vi "E14 BBB Test.vi"(8 "Error In":errorcluster, 11 "Install LV Data":T1={"SSH Session"=refnum, "Status Log"="", "Detailed Log"="", "Credentials"={"Hostname or IP"="192.168.7.2", "Username"="root", "Password"=""}, "Target Info"={"OS Version"="", "CPU"="", "Systemd Version"="", "Internet Access"=FALSE, "Device Type"="", "LV Installed Ver"="", "LV Available Ver"="", "LV Upgrade Available"=FALSE, "Hostname"="", "NIC Info"=[]}, "Reboot Required?"=FALSE}) -> (0 "Error Out":errorcluster, 1 "Status":string, 3 "Install LV Data":T1={"SSH Session"=refnum, "Status Log"="", "Detailed Log"="", "Credentials"={"Hostname or IP"="192.168.7.2", "Username"="root", "Password"=""}, "Target Info"={"OS Version"="", "CPU"="", "Systemd Version"="", "Internet Access"=FALSE, "Device Type"="", "LV Installed Ver"="", "LV Available Ver"="", "LV Upgrade Available"=FALSE, "Hostname"="", "NIC Info"=[]}, "Reboot Required?"=FALSE})   [LabVIEW 2020, in "LMH-LINX.lvlib"]
uses:
  LMH-LINX.lvlib
  Target Management/Install LV Data.ctl
  Target Management/Target Info.ctl
  Target Management/NIC Info.ctl
  Target Management/NIC Mode.ctl
  Toolbox/LMH-Toolbox.lvlib
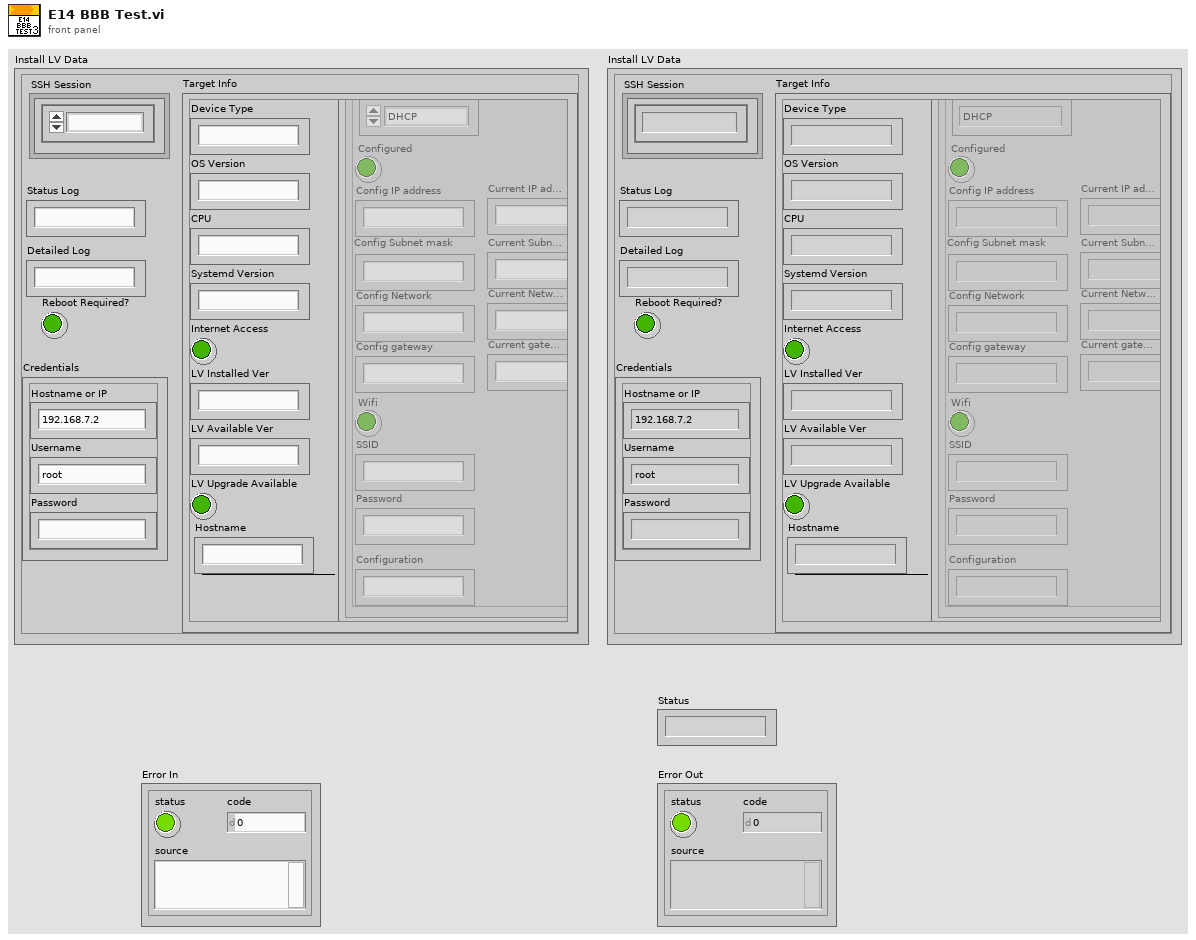
[diagram p1: front panel]
types:
  T1 = typedef "LMH-LINX.lvlib/Install LV Data.ctl" = cluster{"SSH Session":refnum<k1>, "Status Log":string, "Detailed Log":string, "Credentials":cluster{"Hostname or IP":string, "Username":string, "Password":string}, "Target Info":T2, "Reboot Required?":bool}
  T2 = typedef "LMH-LINX.lvlib/Target Info.ctl" = cluster{"OS Version":string, "CPU":string, "Systemd Version":string, "Internet Access":bool, "Device Type":string, "LV Installed Ver":string, "LV Available Ver":string, "LV Upgrade Available":bool, "Hostname":string, "NIC Info":T3[]}
  T3 = typedef "LMH-LINX.lvlib/NIC Info.ctl" = cluster{"Name":string, "NIC Mode":T4, "Configured":bool, "Config IP address":string, "Config Subnet mask":string, "Config Network":string, "Config gateway":string, "Wifi":bool, "SSID":string, "Password":string, "Configuration":string, "Current IP address":string, "Current Subnet mask":string, "Current gateway":string, "Current Network":string}
  T4 = typedef "LMH-LINX.lvlib/NIC Mode.ctl" = enum16{"DHCP", "Static", "Loopback"}
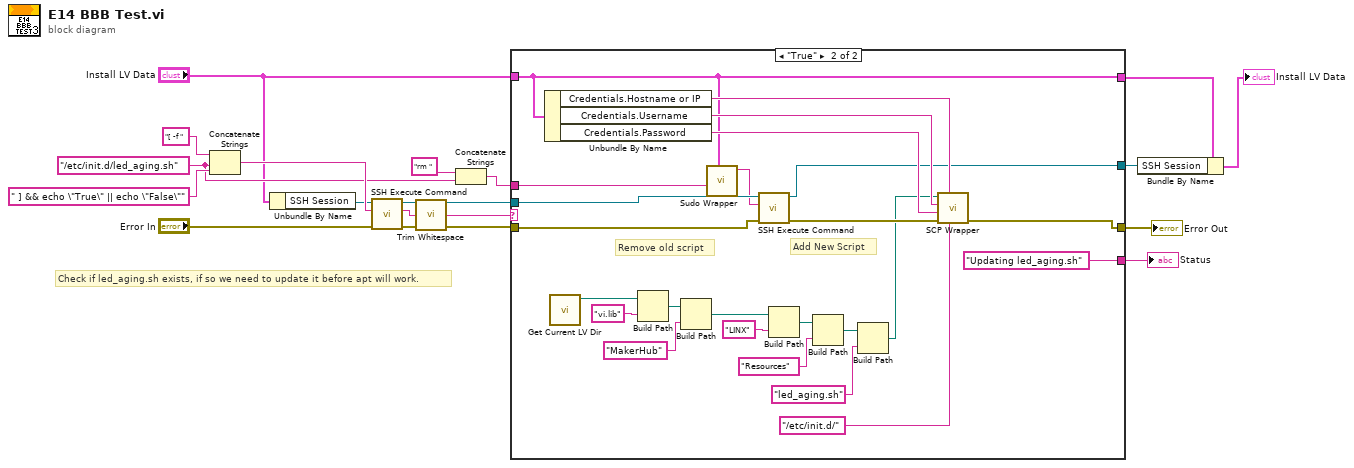
[diagram p0: block diagram]
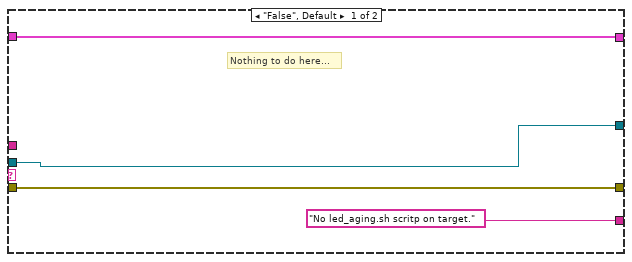
[diagram p2: hidden frame]
diagram:
  w12 = "/etc/init.d/led_aging.sh" ("Command")
  # "Check if led_aging.sh exists, if so we need to update it before apt will work."
  n1 = Concatenate Strings("[ -f " ("Command"), w12, " ] && echo \"True\" || echo \"False\"" ("Command")) -> (w13:string)
  n2 = Unbundle By Name("Install LV Data") -> ("SSH Session"=w8:refnum<k1>)
  n3 = call "SSH Execute Command.vi"("Error In"="Error In", "Command"=w13, "SSH Session"=w8) -> ("Error Out"=w17:errorcluster, "Std Out"=w10:string, "SSH Session"=w16:refnum<k1>)  [unwired: 6 in]
  n4 = call <vilib>:"Trim Whitespace.vi"("string"=w10) -> ("trimmed string"=w9:string)  [unwired: 1 in]
  n5 = Concatenate Strings("rm " ("Command"), w12) -> (w1:string)
  n6 = case shown="\"True\"" w9 {
    tunnel: w17 -> [w22 w46]
    tunnel: w16 -> [w20 w45]
    tunnel: [w22 w28] -> w11
    tunnel: "Install LV Data" -> [w19 w23]
    tunnel: [w19 w23] -> w3
    tunnel: ["No led_aging.sh scritp on target." ("Std Out") "Updating led_aging.sh" ("Std Out")] -> w6
    tunnel: [w20 w27] -> w5
    tunnel: w1 -> [_ w25]
    frame "False", Default {
      # "Nothing to do here..."
    }
    frame "True" {
      # "Remove old script"
      # "Add New Script"
      n7 = Unbundle By Name(w23) -> ("Credentials.Hostname or IP"=w44:string, "Credentials.Username"=w43:string, "Credentials.Password"=w41:string)
      n8 = call "Get Current LV Dir.vi"() -> ("This LV Directory"=w31:path)  [unwired: 10 in, 1 out]
      n9 = Build Path(base path=w31, name or relative path="vi.lib" ("Command")) -> (appended path=w33:path)
      n10 = Build Path(base path=w33, name or relative path="MakerHub" ("Command")) -> (appended path=w34:path)
      n11 = call "Sudo Wrapper.vi"("Install LV Data"=w23, "comand string"=w25) -> ("combined command string"=w24:string)  [unwired: 9 in]
      n12 = call "SSH Execute Command.vi"("Error In"=w46, "Command"=w24, "SSH Session"=w45) -> ("Error Out"=w42:errorcluster, "SSH Session"=w27:refnum<k1>)  [unwired: 6 in, 1 out]
      n13 = Build Path(base path=w34, name or relative path="LINX" ("Command")) -> (appended path=w35:path)
      n14 = Build Path(base path=w35, name or relative path="Resources" ("Command")) -> (appended path=w40:path)
      n15 = Build Path(base path=w40, name or relative path="led_aging.sh") -> (appended path=w30:path)
      n16 = call "SCP Wrapper.vi"("Target Directory"="/etc/init.d/", "Hostname or IP"=w44, "error in (no error)"=w42, "Password"=w41, "Username"=w43, "Local Path"=w30) -> ("error out"=w28:errorcluster)  [unwired: 5 in]
    }
  }
  "Error Out" <- w11
  "Status" <- w6
  n17 = Bundle By Name(cluster=w3, "SSH Session"=w5) -> (→"Install LV Data":T1)
